vi "Random Plot Generator.vi"() -> ()   [LabVIEW 2010]
panel:
  in  "Delay Time (s)":dbl=0.001
  out "Random Numbers":cluster{dbl, dbl}[](graph)
  in  "stop":bool
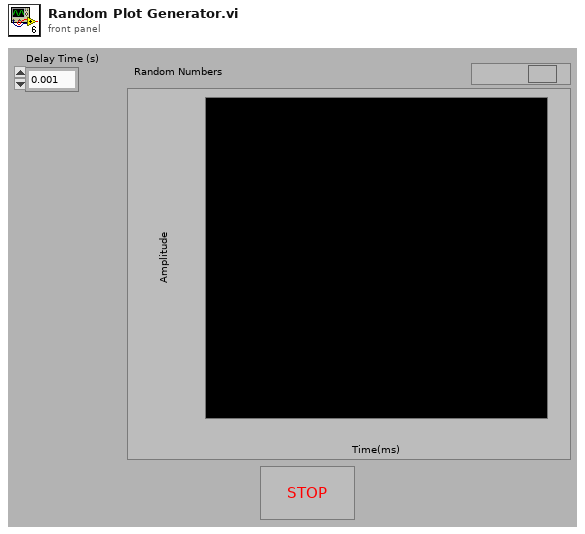
[diagram p1: front panel]
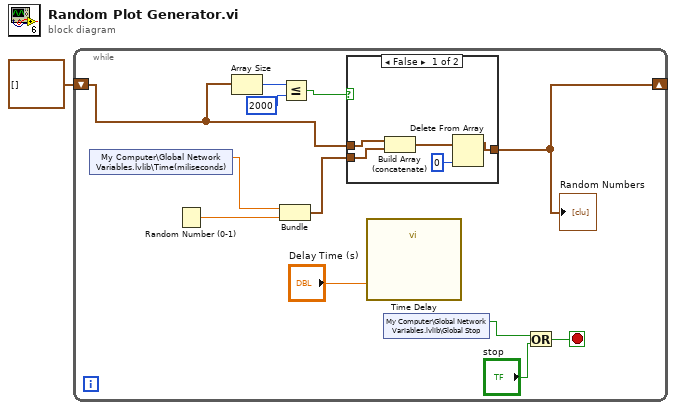
[diagram p0: block diagram]
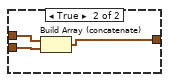
[diagram p2: hidden frame]
diagram:
  n1 = while {
    shift-right: [w8] -> _
    shift-left: cluster{"Double":dbl, "number: 0 to 1":dbl}[] [] -> [w6]
    stop <- w10 stop-if-true
    n2 = shared-variable "My Computer\\Global Network Variables.lvlib\\Time(miliseconds)"() -> (w13:dbl)  [unwired: 1 in, 1 out]
    n3 = Random Number (0-1)() -> (number: 0 to 1=w12:dbl)
    n4 = Array Size(array=w6) -> (size(s)=w4:i32)
    n5 = Bundle("Double"=w13, "number: 0 to 1"=w12) -> (w7:cluster{"Double":dbl, "number: 0 to 1":dbl})  [unwired: 1 in]
    n6 = Less Or Equal?(x=w4, y=2000) -> (x <= y?=w5:bool)
    n7 = case shown="False" w5 {
      tunnel: [w14 w21] -> w8
      tunnel: w6 -> [w18 w20]
      tunnel: w7 -> [w17 w19]
      frame False {
        n8 = Build Array (concatenate)(w18, w17) -> (w15:cluster{"Double":dbl, "number: 0 to 1":dbl}[])
        n9 = Delete From Array(array=w15, index=0) -> (array with subset deleted=w14:cluster{"Double":dbl, "number: 0 to 1":dbl}[])  [unwired: 1 in, 1 out]
      }
      frame True {
        n10 = Build Array (concatenate)(w20, w19) -> (w21:cluster{"Double":dbl, "number: 0 to 1":dbl}[])
      }
    }
    "Random Numbers" <- w8
    n11 = call "Time Delay"("Delay Time (s)"="Delay Time (s)") -> ()  [unwired: 10 in, 1 out]
    n12 = shared-variable "My Computer\\Global Network Variables.lvlib\\Global Stop"() -> (w11:bool)  [unwired: 1 in, 1 out]
    n13 = Or(x=w11, y="stop") -> (x .or. y?=w10:bool)
  }
